vi "IMAQ Interpolation.vi"(10 "Ratio":dbl=2.5, 11 "Image In":T1(plugin-control)) -> (2 "Interpolated Image Size":cluster{"x":i32, "y":i32}, 3 "Interpolated Image":T1(plugin-control))   [LabVIEW 2012, in "LightPipes.lvlib"]
uses:
  LightPipes.lvlib
  <vilib>/gmath/interp.llb/Interpolate 2D (1d X,Y).vi
  <vilib>/gmath/NI_Gmath.lvlib
  <resource>/objmgr/IMAQImage.rc
panel:
  out "y":i32
  out "x":i32
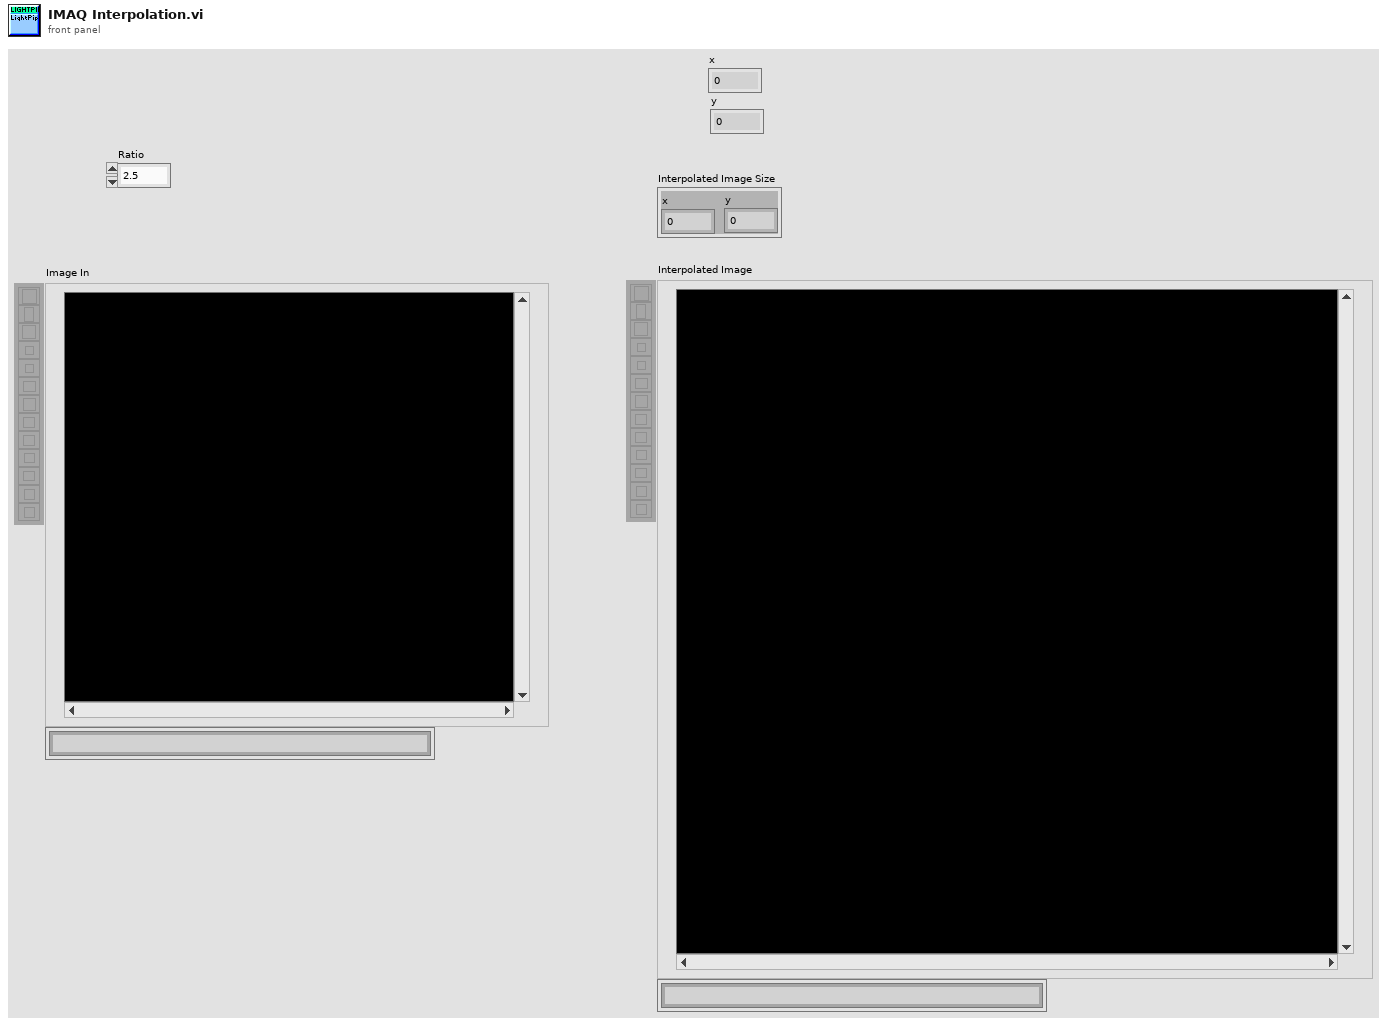
[diagram p1: front panel]
types:
  T1 = typedef "IMAQ Image.ctl" = refnum<image>
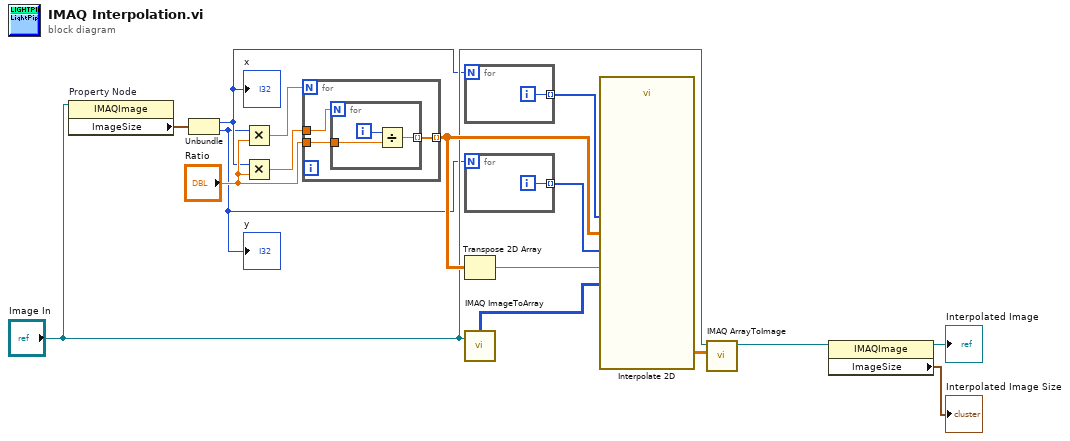
[diagram p0: block diagram]
diagram:
  n1 = property on="Property Node" class="IMAQImage"(reference="Image In") -> ("ImageSize"=w8:cluster{"x":i32, "y":i32})  [unwired: 1 in, 2 out]
  n2 = Unbundle(w8) -> ("x"=w6:i32, "y"=w5:i32)
  "x" <- w6
  "y" <- w5
  n3 = Multiply(x=w5, y="Ratio") -> (x*y=w4:dbl)
  n4 = Multiply(x=w6, y="Ratio") -> (x*y=w3:dbl)
  n5 = for {
    N: w4 -> [_]
    tunnel: "Ratio" -> [w19]
    tunnel: [w18] -> w16 mode=indexing
    tunnel: w3 -> [w17]
    n6 = for {
      N: w17 -> [_]
      tunnel: w19 -> [w21]
      tunnel: [w20] -> w18 mode=indexing
      i -> [w22]
      n7 = Divide(x=w22, y=w21) -> (x/y=w20:dbl)
    }
  }
  n8 = for {
    N: w6 -> [_]
    tunnel: [w23] -> w2 mode=indexing
    i -> [w23]
  }
  n9 = for {
    N: w5 -> [_]
    tunnel: [w24] -> w1 mode=indexing
    i -> [w24]
  }
  n10 = Transpose 2D Array(2D array=w16) -> (transposed array=w15:dbl[][])
  n11 = call "IMAQ ImageToArray"("Image"="Image In") -> ("Image Pixels (U8)"=w14:u8[][])  [unwired: 3 in, 4 out]
  n12 = call-poly <vilib>:"Interpolate 2D.vi"("yi"=w15, "xi"=w16, "Y"=w1, "X"=w2, "Z"=w14) -> ("zi"=w13:dbl[][])  [unwired: 3 in, 3 out]
  n13 = call "IMAQ ArrayToImage"("Image Pixels (U8)"=w13, "Image"="Image In") -> ("Image Out"=w12:T1)  [unwired: 8 in, 1 out]
  n14 = property class="IMAQImage"(reference=w12) -> (reference out=→"Interpolated Image":T1, "ImageSize"=→"Interpolated Image Size":cluster{"x":i32, "y":i32})  [unwired: 1 in, 1 out]
